vi "Streamlined FPGA--130415-3.vi"() -> ()   [LabVIEW 2009]
uses:
  <vilib>/eio/EIONode/EIONode.xnode
  <vilib>/rvi/eio/nirviEIOImplementation/nirviEIOImplementation.xnode
  <vilib>/rvi/eio/common/nirviEmuTemplateMethod_noerrors.vi
  <vilib>/rvi/eio/common/nirviEmuClasses.ctl
  Instance           3 24Saved   Streamlined FPGA .vi
  Instance           4 24Saved   Streamlined FPGA .vi
  Instance           5 24Saved   Streamlined FPGA .vi
  Instance           2 24Saved   Streamlined FPGA .vi
  <vilib>/rvi/DataTransferAndStorage/Container/XNode/niFpgaContainer.xnode
  <vilib>/rvi/interface/RandomDataEmulation/niFpgaRandomDataHandleErrors.vi
  <vilib>/rvi/interface/RandomDataEmulation/nirviRandomDataFPGAFIFO.vi
  <vilib>/rvi/DataTransferAndStorage/Container/Common/niFpgaContainerMethod.ctl
  <vilib>/rvi/DataTransferAndStorage/Container/Common/niFpgaTransferTypeControl.ctl
panel:
  in  "Array 2":cluster{"[0]":i32, "[1]":i32, "[2]":i32}[](array[cluster])=[{"[0]"=3276800, "[1]"=1000, "[2]"=1}, {"[0]"=3276800, "[1]"=1000, "[2]"=1}, {"[0]"=0, "[1]"=0, "[2]"=0}, {"[0]"=0, "[1]"=0, "[2]"=1}]
  in  "window size":i32
  out "sort!":bool
  in  "Maximum Width":i16
  in  "Maximum Height":i16
  in  "trigger on all":bool
  out "sort pulse":i16
  in  "Baselines":i16[](array[numeric])=[0, 0, 0, 0]
  in  "Sb":i8(ring)=1 items=["PMT1", "PMT2", "PMT3", "PMT4"]
  in  "Sa":i8(ring) items=["PMT1", "PMT2", "PMT3", "PMT4"]
  in  "Sort Case":i8(ring)=1 items=["FP", "Magnitude"]
  out "Full 2":bool
  in  "sort?":bool
  out "Drop counter":u32
  out "sort counter":u32
  in  "PMT to detect drops on":u8
  in  "Minimum Height":i16
  in  "Minimum Width":i16
  in  "Ticks between acquires (Ticks)":u32=200
  in  "Gain 1":i16(slide) scale=-32767.0..32767.0
  in  "Gain 2":i16(slide) scale=-32767.0..32767.0
  in  "Gain 3":i16(slide) scale=-32767.0..32767.0
  in  "Gain 4":i16(slide) scale=-32767.0..32767.0
  in  "amplitude":i16
  in  "1/Frequency \n(ticks)":u32
  in  "Burst \nCycles":i32
  in  "delay [us]":u32=20 min=1 max=8000
  # "Acquisition and Detection"
  # "FP and Sorting Parameters"
  # "Sorting Pulse\nGenerator"
  # "Events"
  # "PMT Controls"
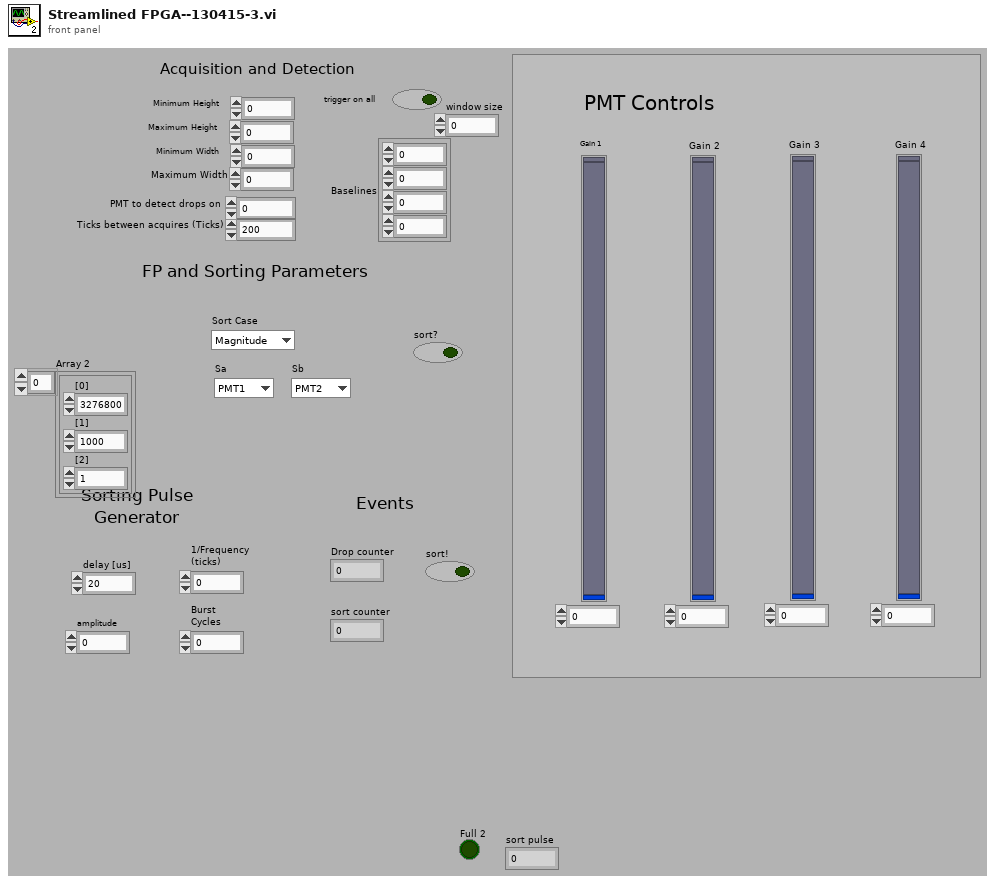
[diagram p1: front panel]
types:
  T1 = typedef "nirviEmuClasses.ctl" = enum16{"IO Read", "IO Write", "Method", "Property Read", "Property Write"}
  T2 = typedef "niFpgaContainerMethod.ctl" = enum16{"Write", "Read", "Clear", "Get Number of Elements to Write", "Get Number of Elements to Read", "Enable", "Disable", "Flush and Disable", "Get Stream State"}
  T3 = typedef "niFpgaTransferTypeControl.ctl" = enum16{"Target-Scoped", "Host to Target - DMA", "Target to Host - DMA", "Peer to Peer Reader", "Peer to Peer Writer", "Bidirectional"}
  T4 = cluster{bool, "max":i16[], "sum":i32[], "time inside":i32, "time outside":i32, "timeoutside-1":i32}
  T5 = cluster{"maxes":i16[], "sums":i32[], "time inside":i32, "time outside":i32}
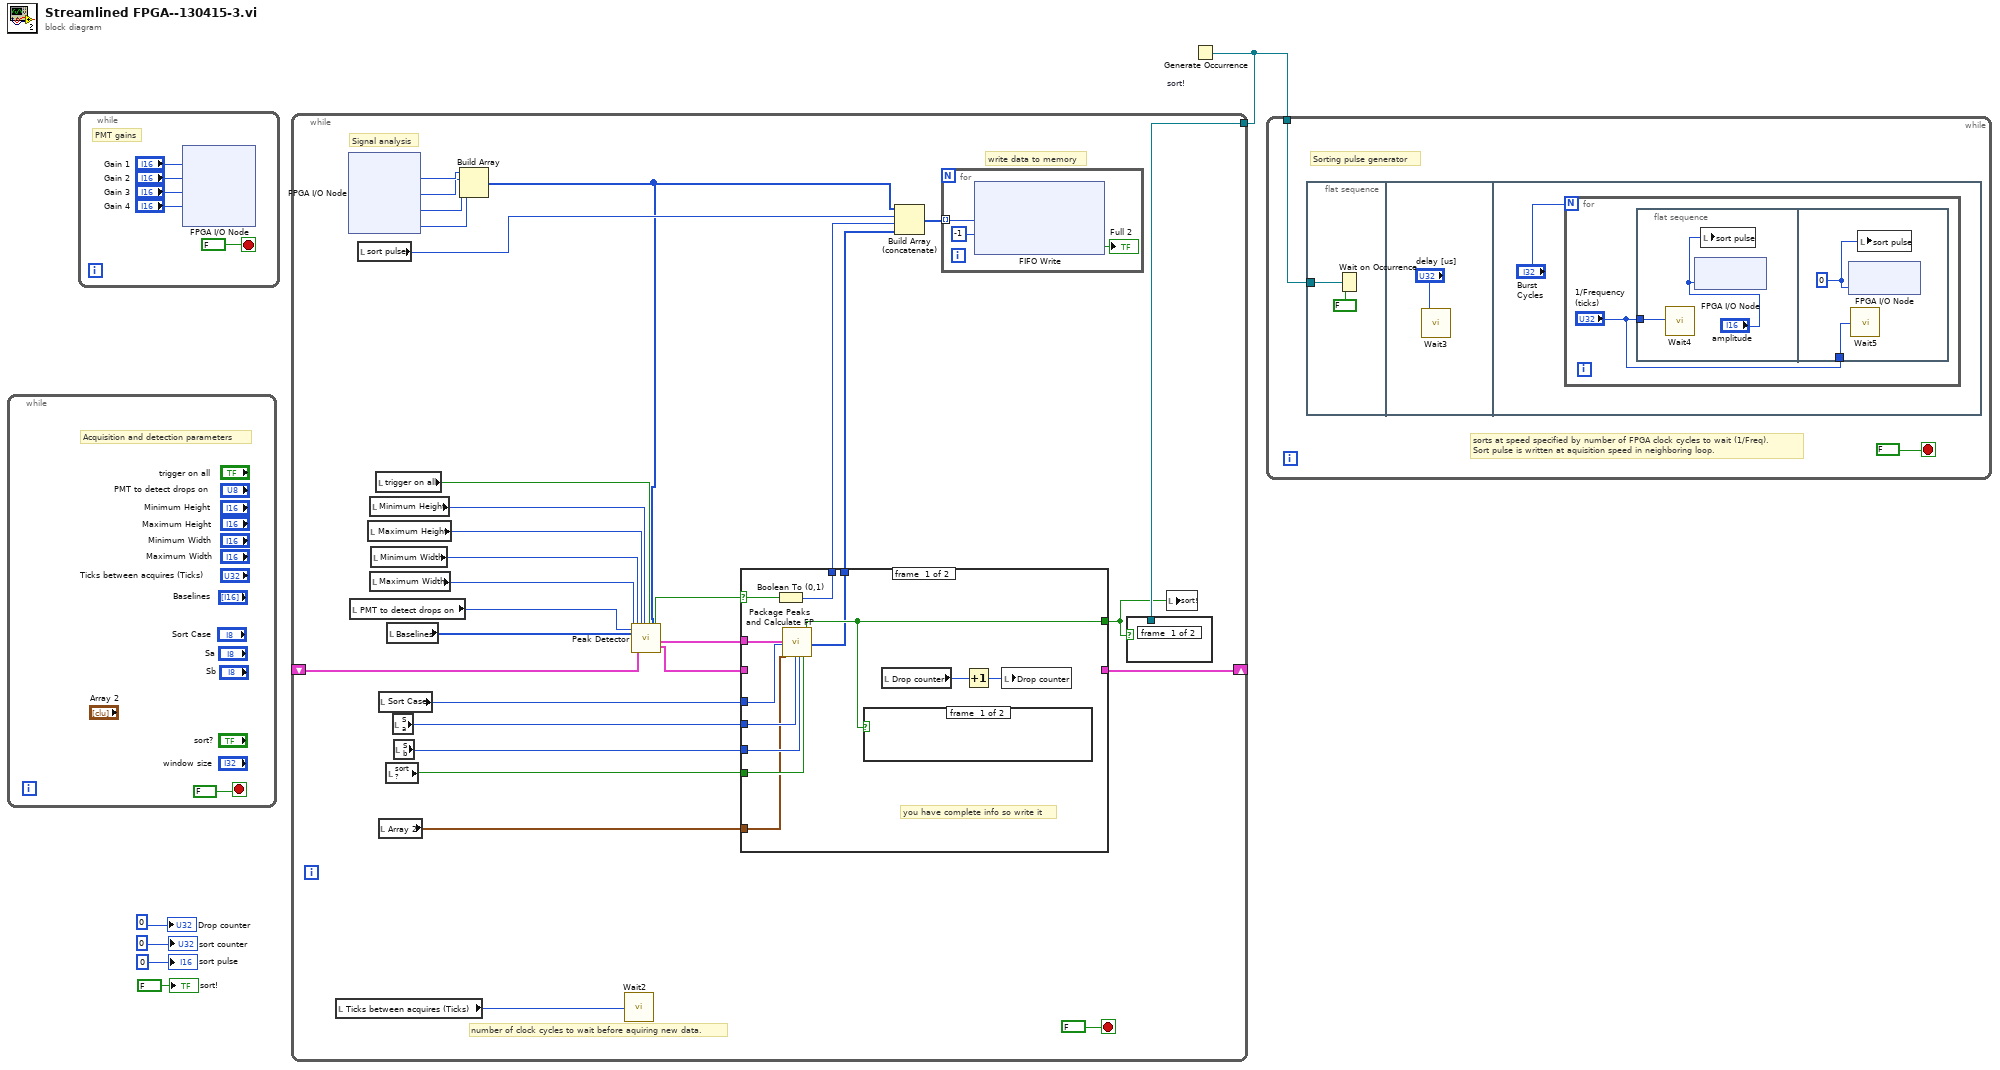
[diagram p0: block diagram]
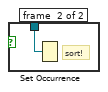
[diagram p2: hidden frame]
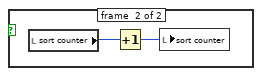
[diagram p3: hidden frame]
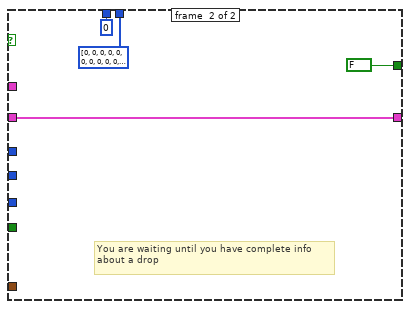
[diagram p4: hidden frame]
diagram:
  n1 = while {
    stop <- FALSE stop-if-true
    # "Acquisition and detection parameters"
  }
  n2 = while {
    stop <- FALSE stop-if-true
    # "PMT gains"
    n3 = xnode "FPGA I/O Node"("AO0"="Gain 1", "AO1"="Gain 2", "AO2"="Gain 3", "AO3"="Gain 4") -> ()  [unwired: 4 in, 4 out]
  }
  n4 = Generate Occurrence "sort!"() -> (w5:refnum<k4>)
  n5 = while {
    shift-right: [w84] -> _
    shift-left: _ -> [w71]
    tunnel: w5 -> [w69]
    stop <- FALSE stop-if-true
    # "number of clock cycles to wait before aquiring new data."
    # "Signal analysis"
    # "write data to memory"
    n6 = local read "Ticks between acquires (Ticks)"() -> (w79:u32)
    n7 = xnode "FPGA I/O Node"() -> ("AI0"=w83:i16, "AI1"=w82:i16, "AI2"=w81:i16, "AI3"=w80:i16)  [unwired: 4 in, 4 out]
    n8 = local read "PMT to detect drops on"() -> (w61:u8)
    n9 = local read "sort pulse"() -> (w68:i16)
    n10 = local read "Maximum Height"() -> (w64:i16)
    n11 = local read "Minimum Height"() -> (w65:i16)
    n12 = local read "Maximum Width"() -> (w62:i16)
    n13 = local read "Minimum Width"() -> (w63:i16)
    n14 = local read "trigger on all"() -> (w70:bool)
    n15 = local read "Sort Case"() -> (w78:i8)
    n16 = local read "Array 2"() -> (w56:cluster{"[0]":i32, "[1]":i32, "[2]":i32}[])
    n17 = local read "sort?"() -> (w75:bool)
    n18 = local read "Baselines"() -> (w60:i16[])
    n19 = local read "Sa"() -> (w77:i8)
    n20 = local read "Sb"() -> (w76:i8)
    n21 = Build Array(w83, w82, w81, w80) -> (w57:i16[])
    n22 = call "Wait2"("Count(Ticks)"=w79) -> ()  [unwired: 1 out]
    n23 = call "Peak Detector.vi"("Maximum Width"=w62, "PMT to trigger on (0,1,2,3)"=w61, "Baselines"=w60, "Minimum Width"=w63, "shifts in"=w71, "Maximum Height"=w64, "Minimum Height"=w65, "trigger on all"=w70, "s1,s2,s3,s4"=w57) -> ("peak complete?"=w74:bool, "shifts out"=w72:T4, "peaks data"=w73:T5)  [unwired: 16 in]
    n24 = case shown="True" w74 {
      selector: w74 -> [w196 _]
      tunnel: [_ w207] -> w84
      tunnel: [w194 FALSE ("sort!")] -> w59
      tunnel: w78 -> [w192 _]
      tunnel: w77 -> [w200 _]
      tunnel: w76 -> [w199 _]
      tunnel: w75 -> [w198 _]
      tunnel: w72 -> [_ w207]
      tunnel: w73 -> [w197 _]
      tunnel: [w195 i16 0] -> w66
      tunnel: [w193 i32[] [0, 0, 0, 0, 0, 0, 0, 0, 0, 0, 0, 0] ("M1,M2,M3,M4,S1,S2,S3,S4,Tin,Tout,FP")] -> w58
      tunnel: w56 -> [w191 _]
      frame #0 {
        # "you have complete info so write it"
        n25 = Boolean To (0,1)(Boolean=w196) -> (0, 1=w195:i16)
        n26 = call "Package Peaks and Calculate FP.vi"("peaks data"=w197, "Sort Case"=w192, "Array 2"=w191, "Sa"=w200, "Sb"=w199, "sort?"=w198) -> ("sort!"=w194:bool, "M1,M2,M3,M4,S1,S2,S3,S4,Tin,Tout,FP,Sort?"=w193:i32[])  [unwired: 16 in, 4 out]
        n27 = case shown="True" w194 {
          frame #0 {
          }
          frame #1 {
            n28 = local read "sort counter"() -> (w204:u32)
            n29 = Increment(x=w204) -> (x+1=w203:u32)
            n30 = local write "sort counter"(w203) -> ()
          }
        }
        n31 = local read "Drop counter"() -> (w202:u32)
        n32 = Increment(x=w202) -> (x+1=w201:u32)
        n33 = local write "Drop counter"(w201) -> ()
      }
      frame #1 {
        # "You are waiting until you have complete info about a drop"
      }
    }
    n34 = Build Array (concatenate)(w57, w68, w66, w58) -> (w67:i32[])
    n35 = for {
      tunnel: w67 -> [w89] mode=indexing
      n36 = xnode ("FIFO Write")("Element"=w89, "Timeout"=-1) -> ("Timed Out?"=→"Full 2":bool)  [unwired: 1 in, 1 out]
    }
    n37 = case shown="True" w59 {
      tunnel: w69 -> [_ w86]
      frame #0 {
      }
      frame #1 {
        # "sort!"
        n38 = Set Occurrence(w86) -> ()
      }
    }
    n39 = local write "sort!"(w59) -> ()
  }
  n40 = while {
    tunnel: w5 -> [w209]
    stop <- FALSE stop-if-true
    # "sorts at speed specified by number of FPGA clock cycles to wait (1/Freq).\nSort pulse is written at aquisition speed in neighboring loop."
    # "Sorting pulse generator"
    n41 = flat-sequence {
      tunnel: w209 -> [w211]
      frame #0 {
        n42 = Wait on Occurrence(1:FALSE ("ignore previous (T)"), 2:w211) -> ()  [unwired: 1 in, 1 out]
      }
      frame #1 {
        n43 = call "Wait3"("Count(uSec)"="delay [us]") -> ()  [unwired: 1 out]
      }
      frame #2 {
        n44 = for {
          N: "Burst \nCycles" -> [_]
          n45 = flat-sequence {
            tunnel: "1/Frequency \n(ticks)" -> [w217]
            tunnel: "1/Frequency \n(ticks)" -> [w230]
            frame #0 {
              n46 = call "Wait4"("Count(Ticks)"=w217) -> ()  [unwired: 1 out]
              n47 = xnode "FPGA I/O Node"("AO4"="amplitude") -> ()  [unwired: 1 in, 1 out]
              n48 = local write "sort pulse"("amplitude") -> ()
            }
            frame #1 {
              w229 = i16 0 ("sort pulse")
              n49 = xnode "FPGA I/O Node"("AO4"=w229) -> ()  [unwired: 1 in, 1 out]
              n50 = call "Wait5"("Count(Ticks)"=w230) -> ()  [unwired: 1 out]
              n51 = local write "sort pulse"(w229) -> ()
            }
          }
        }
      }
    }
  }
  "sort counter" <- u32 0 ("event counter")
  "Drop counter" <- u32 0 ("Drop counter")
  "sort pulse" <- i16 0 ("event counter")
  "sort!" <- FALSE ("sort!")
